vi "Untitled 5 (SubVI).vi"(7 "Section":string, 8 "Error in":errorcluster caption="Error in (no error)", 11 "String might with variables":string) -> (0 "Error out":errorcluster, 3 "String out":string)   [LabVIEW 2017]
uses:
  <userlib>/_NEVSTOP/Communicable State Machine(CSM)/Communicable State Machine.lvlib
  INI-Static-Variable-Support/INI-Static-Variable-Support.lvlib
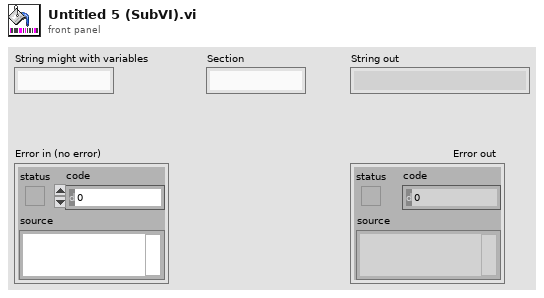
[diagram p1: front panel]
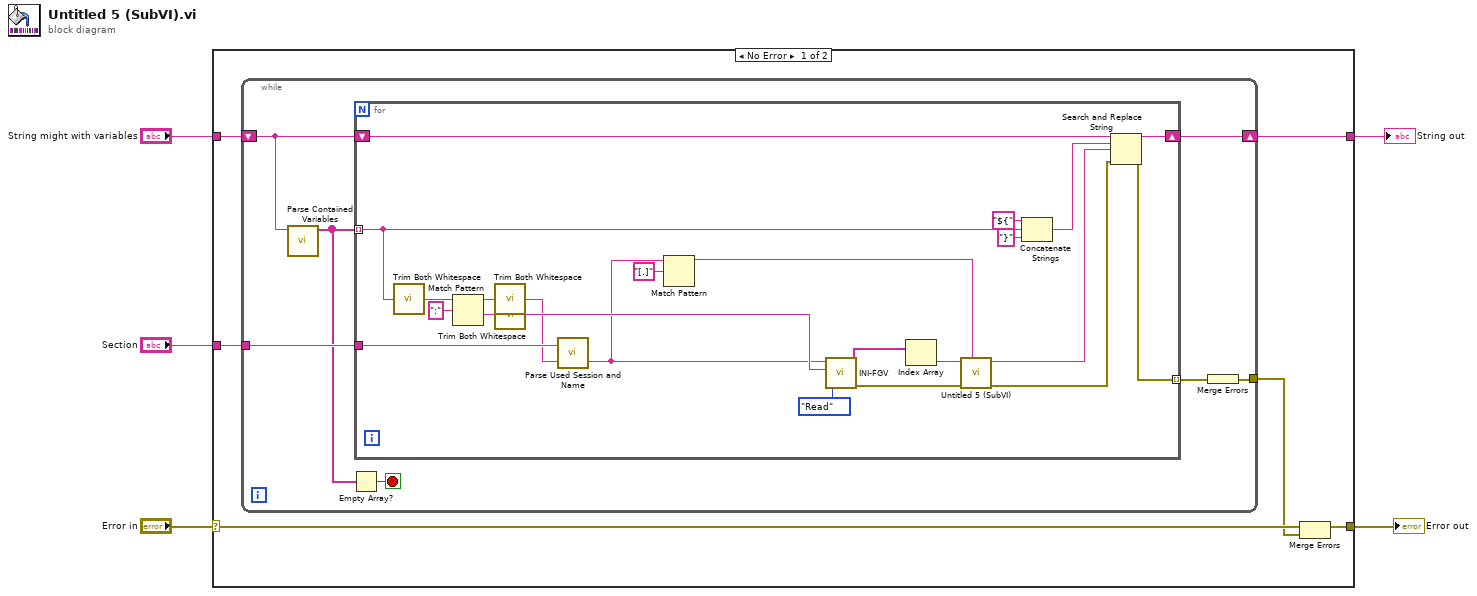
[diagram p0: block diagram]
diagram:
  n1 = case shown="No Error" "Error in" {
    selector: "Error in" -> [w8 w43]
    tunnel: [w11 w42] -> w5
    tunnel: "Section" -> [w10 _]
    tunnel: "String might with variables" -> [w9 w42]
    tunnel: [w7 w43] -> w1
    frame No Error {
      n2 = while {
        shift-right: [w17] -> w11
        shift-left: w9 -> [w15]
        tunnel: w10 -> [w18]
        tunnel: [w12] -> w6
        stop <- w16 stop-if-true
        n3 = call "Parse Contained Variables.vi"("String"=w15) -> ("Contained Variables"=w14:string[])  [unwired: 10 in]
        n4 = Empty Array?(array=w14) -> (empty?=w16:bool)
        n5 = for {
          tunnel: w14 -> [w34] mode=indexing
          shift-right: [w38] -> w17
          shift-left: w15 -> [w39]
          tunnel: [w36] -> w13 mode=indexing
          tunnel: w18 -> [w35]
          n6 = call <userlib>:"Trim Both Whitespace.vi"("string"=w34) -> ("trimmed string"=w24:string)  [unwired: 1 in]
          n7 = Match Pattern(string=w24, regular expression=":") -> (before substring=w32:string, after substring=w31:string)  [unwired: 1 in, 2 out]
          n8 = call <userlib>:"Trim Both Whitespace.vi"("string"=w32) -> ("trimmed string"=w29:string)  [unwired: 1 in]
          n9 = call <userlib>:"Trim Both Whitespace.vi"("string"=w31) -> ("trimmed string"=w30:string)  [unwired: 1 in]
          n10 = call "Parse Used Session and Name.vi"("name"=w29, "Section Name(\"\" as Default)"=w35) -> ("used name"=w28:string)  [unwired: 1 in]
          n11 = Match Pattern(string=w28, regular expression="[.]") -> (before substring=w23:string)  [unwired: 1 in, 3 out]
          n12 = call "INI-FGV.vi"("Enum"=enum16{"Read", "Write", "Sync"}."Read", ">> Default Value >>"=w30, ">> Variable Name >>"=w28) -> ("error out"=w20:errorcluster, "Array"=w26:string[])  [unwired: 5 in, 2 out]
          n13 = Index Array(array=w26) -> (element=w22:string)  [unwired: 1 in]
          n14 = call "Untitled 5 (SubVI).vi"("Section"=w23, "Error in"=w20, "String might with variables"=w22) -> ("Error out"=w19:errorcluster, "String out"=w21:string)  [unwired: 7 in]
          n15 = Concatenate Strings("${" ("regular expression"), w34, "}" ("regular expression")) -> (w37:string)
          n16 = Search and Replace String(input string=w39, search string=w37, replace string=w21, error in=w19) -> (result string=w38:string, error out=w36:errorcluster)  [unwired: 4 in, 2 out]
        }
        n17 = Merge Errors(w13) -> (w12:errorcluster)
      }
      n18 = Merge Errors(w8, w6) -> (w7:errorcluster)
    }
    frame Error {
    }
  }
  "String out" <- w5
  "Error out" <- w1
